vi "Get Process VI Actions.vi"(8 "error in (no error)":errorcluster {"code" format="Error %.0f"}, 11 "VIDoc Printer In":refnum<class "VIDoc Printer.lvclass">) -> (0 "error out":errorcluster {"code" format="Error %.0f"}, 2 "Process VI Actions":T1[](array[typedef]), 3 "VIDoc Printer Out":refnum<class "VIDoc Printer.lvclass">)   [LabVIEW 2023, in "VIDoc Printer.lvlib" / "VIDoc Printer.lvclass"]
uses:
  VIDoc Printer.lvclass
  Controls/Process VI Enum.ctl
  VIDoc Printer.lvclass/VIDoc Printer.ctl
  Get VI Settings - Memory.vi
  Get VI Settings - By Folder.vi
  Get VI Settings - By Tree.vi
  Get VI Settings - By List.vi
  Get VI Settings - List Detail Level.vi
  Get VI Settings - Methods.vi
  Get VI Settings - Methods Detail Level.vi
  Get VI Settings - Method Options - Front Panels.vi
  Get VI Settings - Method Options - Options.vi
  Get VI Settings - Method Options - Controls.vi
  Get VI Settings - Controls Detail Level.vi
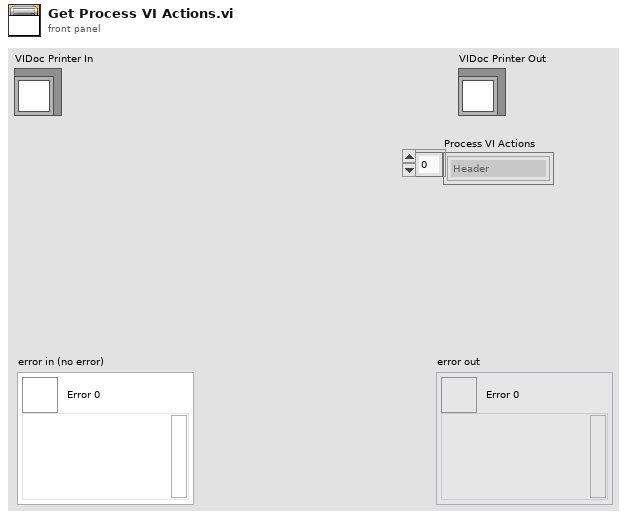
[diagram p1: front panel]
types:
  T1 = typedef "VIDoc Printer.lvlib/VIDoc Printer.lvclass/Process VI Enum.ctl" = enum16{"Header", "Memory", "By Folder", "By Tree", "By List", "Method Details", "FP"}
  T2 = typedef "VIDoc Printer.lvlib/Printer Settings.lvclass/Detail Level Enum.ctl" = enum16{"None", "Minimal", "Standard", "Full"}
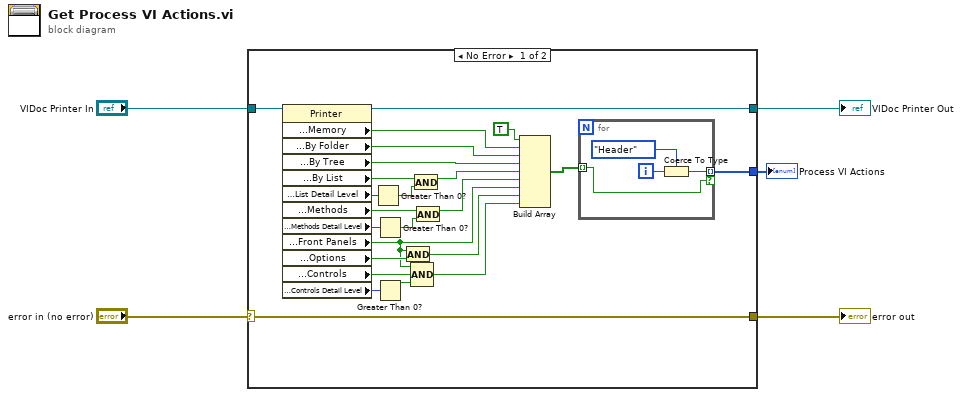
[diagram p0: block diagram]
diagram:
  n1 = case shown="No Error" "error in (no error)" {
    selector: "error in (no error)" -> [w29 w35]
    tunnel: [w29 w35] -> w4
    tunnel: [w21 w34] -> w2
    tunnel: "VIDoc Printer In" -> [w22 w34]
    tunnel: [w19 _] -> w1
    frame No Error {
      n2 = property class="Printer"(reference=w22) -> (reference out=w21:refnum<class "VIDoc Printer.lvclass">, "Properties:Settings:VI Members:Memory"=w27:bool, "Properties:Settings:VI Members:By Folder"=w26:bool, "Properties:Settings:VI Members:By Tree"=w25:bool, "Properties:Settings:VI Members:By List"=w24:bool, "Properties:Settings:VI Members:List Detail Level"=w17:T2, "Properties:Settings:VI Members:Methods"=w23:bool, "Properties:Settings:VI Members:Methods Detail Level"=w18:T2, "Properties:Settings:VI Members:Front Panels"=w10:bool, "Properties:Settings:VI Members:Options"=w12:bool, "Properties:Settings:VI Members:Controls"=w9:bool, "Properties:Settings:VI Members:Controls Detail Level"=w7:T2)  [unwired: 1 in, 1 out]
      n3 = Greater Than 0?(x=w17) -> (x > 0?=w15:bool)
      n4 = Greater Than 0?(x=w18) -> (x > 0?=w13:bool)
      n5 = Greater Than 0?(x=w7) -> (x > 0?=w8:bool)
      n6 = And(x=w10, y=w12) -> (x .and. y?=w11:bool)
      n7 = And(x=w24, y=w15) -> (x .and. y?=w16:bool)
      n8 = Compound Arithmetic op=AND(w10, w9, w8) -> (w6:bool)
      n9 = And(x=w23, y=w13) -> (x .and. y?=w14:bool)
      n10 = Build Array(TRUE ("element"), w27, w26, w25, w16, w14, w10, w11, w6) -> (w20:bool[])
      n11 = for {
        tunnel: w20 -> [w30] mode=indexing
        tunnel: [w31] -> w19 mode=indexing if=w30
        i -> [w32]
        n12 = Coerce To Type(0:w32, 1:Process_VI_Enum."Header") -> (2:w31:T1)
      }
    }
    frame Error {
    }
  }
  "error out" <- w4
  "VIDoc Printer Out" <- w2
  "Process VI Actions" <- w1
